vi "pump_GB01.vi"() -> ()   [LabVIEW 2018]
panel:
  out "Numeric 2":i32=13
  in  "stop":bool
  in  "RUN":bool
  in  "Setting Tab":enum32{"Pump", "OTO"}(tab)
  in  "VISA resource name":refnum<visa-resource-name>="COM3"
  in  "rate (ml/min)":dbl=0.001
  in  "Each Pumping Time":u32=1000
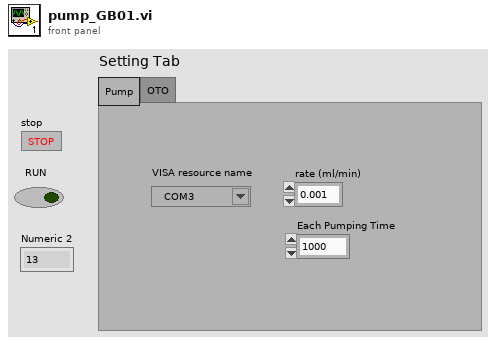
[diagram p1: front panel]
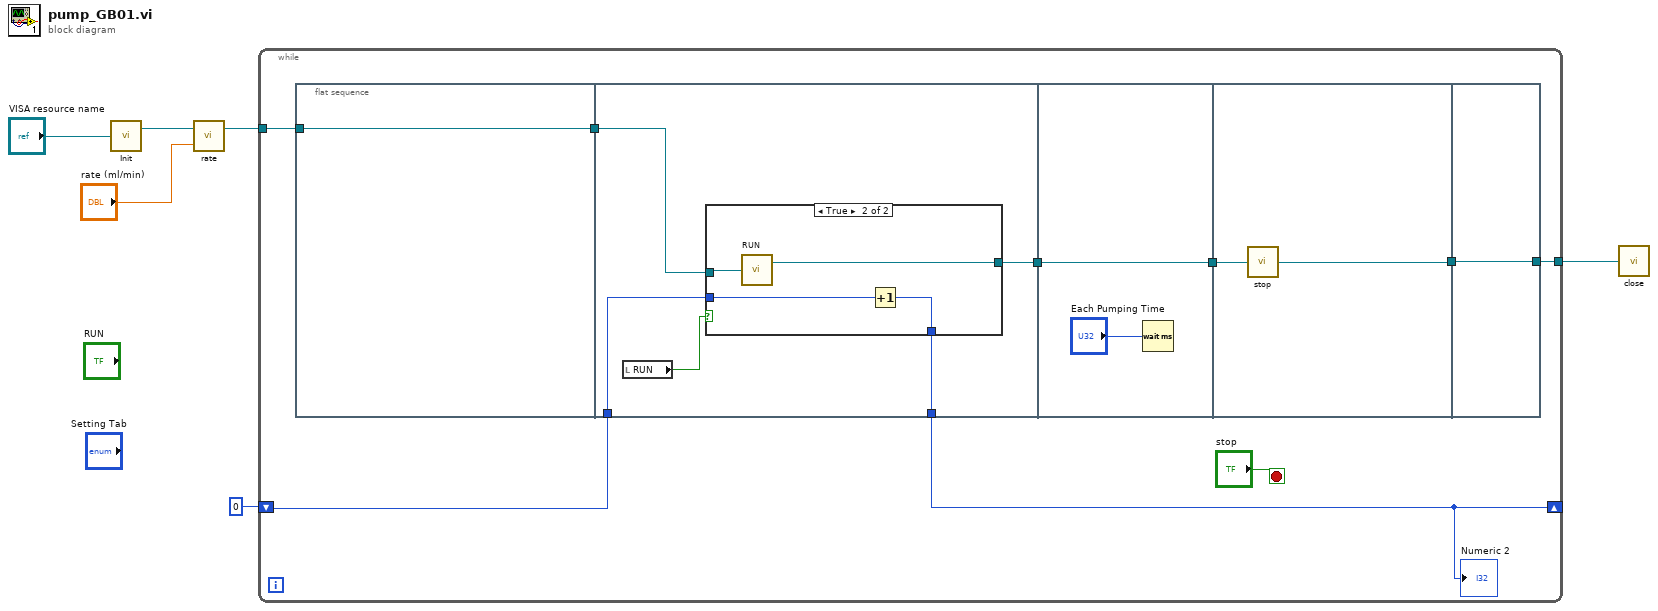
[diagram p0: block diagram]
diagram:
  n1 = call <instrlib>:"Init.vi"("VISA resource name"="VISA resource name") -> ("VISA resource name out"=w5:refnum<visa-resource-name>)  [unwired: 1 out]
  n2 = call <instrlib>:"rate.vi"("rate"="rate (ml/min)", "VISA resource name"=w5) -> ("VISA resource name out"=w3:refnum<visa-resource-name>)  [unwired: 1 out]
  n3 = while {
    tunnel: w3 -> [w13]
    shift-right: [w8] -> _
    shift-left: 0 -> [w9]
    tunnel: [w7] -> w1
    stop <- "stop" stop-if-true
    n4 = flat-sequence {
      tunnel: [w16] -> w15
      tunnel: w13 -> [w16]
      tunnel: w15 -> [w21]
      tunnel: [w20] -> w11
      tunnel: w9 -> [w18]
      tunnel: [w17] -> w8
      tunnel: [w29] -> w12
      tunnel: w11 -> [w29]
      tunnel: w12 -> [w31]
      tunnel: [w30] -> w10
      tunnel: w10 -> [w32]
      tunnel: [w32] -> w7
      frame #0 {
      }
      frame #1 {
        n5 = local read "RUN"() -> (w19:bool)
        n6 = case shown="True" w19 {
          tunnel: w21 -> [w23 w27]
          tunnel: [w23 w26] -> w20
          tunnel: w18 -> [w22 w25]
          tunnel: [w22 w24] -> w17
          frame False {
          }
          frame True {
            n7 = call <instrlib>:"RUN.vi"("VISA resource name"=w27) -> ("VISA resource name out"=w26:refnum<visa-resource-name>)  [unwired: 1 out]
            n8 = Increment(x=w25) -> (x+1=w24:i32)
          }
        }
      }
      frame #2 {
        n9 = Wait (ms)(milliseconds to wait="Each Pumping Time") -> ()  [unwired: 1 out]
      }
      frame #3 {
        n10 = call <instrlib>:"stop.vi"("VISA resource name"=w31) -> ("VISA resource name out"=w30:refnum<visa-resource-name>)
      }
      frame #4 {
      }
    }
    "Numeric 2" <- w8
  }
  n11 = call <instrlib>:"close.vi"("VISA resource name"=w1) -> ()
